vi "Send Cmd To Stimulator_v0.1.vi"(0 "Stimulator In":T2={"Log File In"=refnum, "Stimulator In"="", "Stimulator Mode"="", "Log Data"=FALSE, "Doublet/Triplet  Interval"=0.0, "Stim Frequency"=40.0, "N-Factor"=0, "Active Channels"=[TRUE, TRUE, TRUE, TRUE, TRUE], "Low-Frequency Channels"=[FALSE, FALSE, FALSE, FALSE, FALSE], "Stimulator State"=enum."Closed", "Mode Array"=[], "Current Array"=[], "Pulse Duration Array"=[], "VISA Timeout"=50}, 1 "Command":T1, 3 "error in (no error)":errorcluster) -> (4 "Numeric Response":u8, 5 "Stimulator Out":T2={"Log File In"=refnum, "Stimulator In"="", "Stimulator Mode"="", "Log Data"=FALSE, "Doublet/Triplet  Interval"=0.0, "Stim Frequency"=40.0, "N-Factor"=0, "Active Channels"=[TRUE, TRUE, TRUE, TRUE, TRUE], "Low-Frequency Channels"=[FALSE, FALSE, FALSE, FALSE, FALSE], "Stimulator State"=enum."Closed", "Mode Array"=[], "Current Array"=[], "Pulse Duration Array"=[], "VISA Timeout"=50}, 6 "Command":T1, 7 "Log Entry":string, 8 "error out":errorcluster)   [LabVIEW 2019]
uses:
  Controls/Stimulator Cluster.ctl
  Controls/Stimulator Mode.ctl
  Version 2/Data Type Defs/Pulse Mode (array).ctl
  Controls/Stim Current Array.ctl
  Controls/Pulse Duration Array.ctl
  Bits Library/Get Bit (U8).vi
  Bits Library/Change Bit (U8).vi
  Bits Library/Bits.lvlib
panel:
  out "Write Error":errorcluster
  out "Bytes written":u32
  out "Bytes read":u32
  out "Read Error":errorcluster
  out "resulting string":string
  out "string":string
  out "hex integer string":string
  out "Number Out":u8 format="%.0x"
  out "appended array":bool[](array[boolean])
  out "element":u8 format="%0d"
  out "unsigned byte array 2":u8[](array[numeric]) format="%08b"
  out "Bytes available":u32
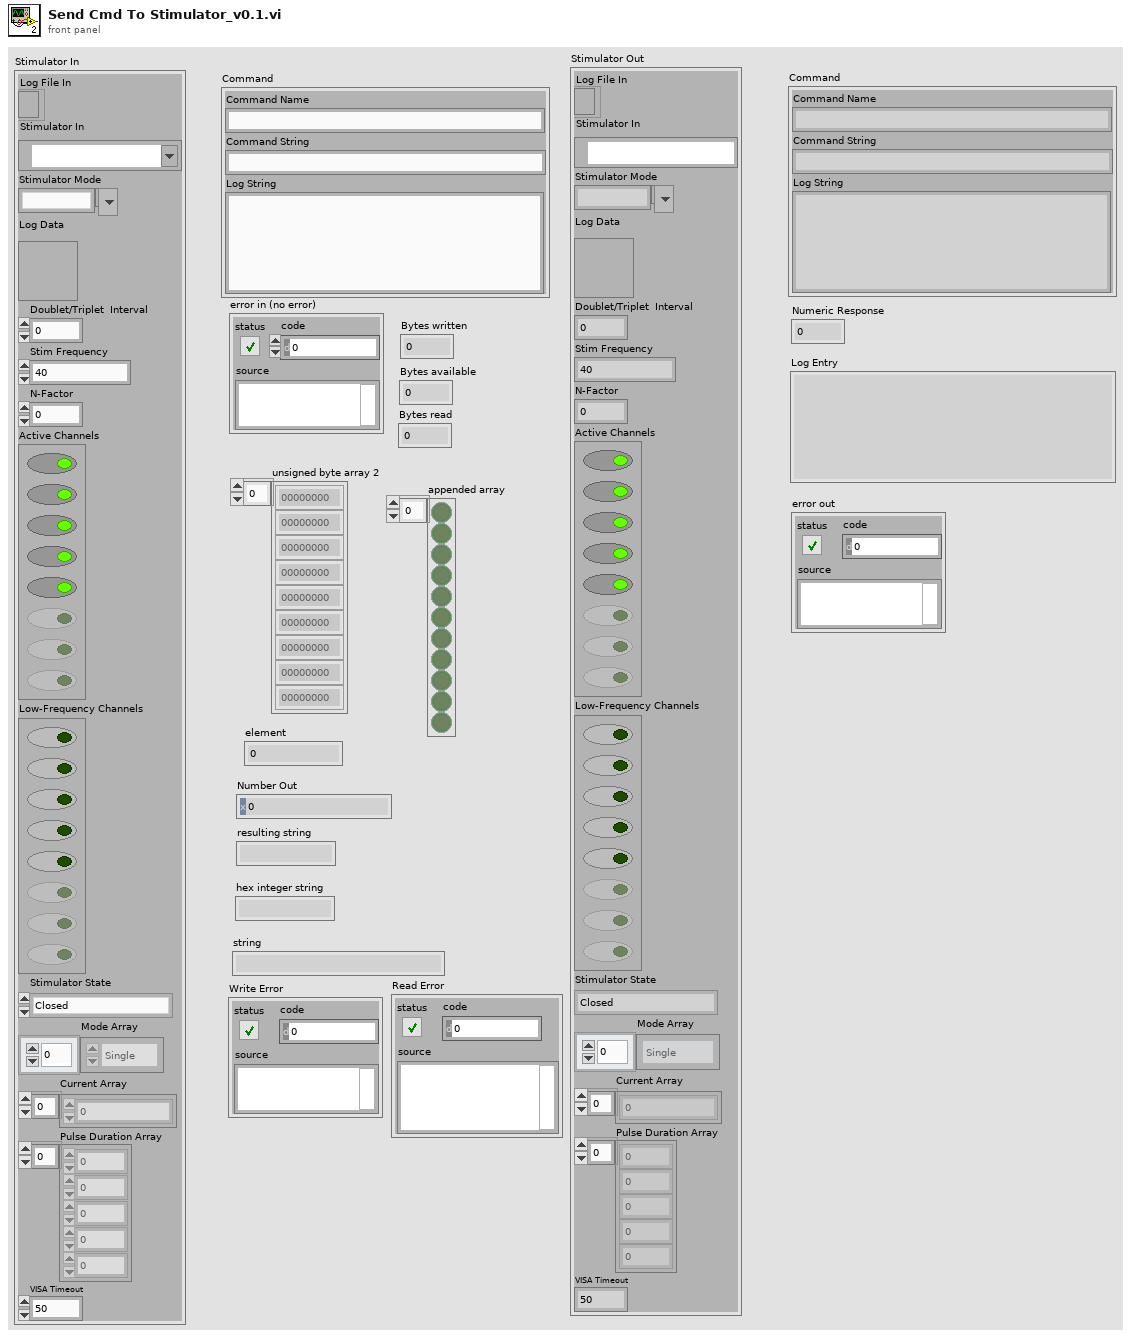
[diagram p1: front panel]
types:
  T1 = cluster{"Command Name":string, "Command String":string, "Log String":string}
  T2 = typedef "Stimulator Cluster.ctl" = cluster{"Log File In":refnum<file>, "Stimulator In":refnum<visa-resource-name>, "Stimulator Mode":T3, "Log Data":bool, "Doublet/Triplet  Interval":dbl, "Stim Frequency":dbl, "N-Factor":u8, "Active Channels":bool[], "Low-Frequency Channels":bool[], "Stimulator State":enum16{"Closed", "Open", "Initialized", "Stimulating"}, "Mode Array":T4, "Current Array":T5, "Pulse Duration Array":T6, "VISA Timeout":u32}
  T3 = typedef "Stimulator Mode.ctl" = string
  T4 = typedef "Pulse Mode (array).ctl" = enum16{"Single", "Doublet", "Triplet"}[]
  T5 = typedef "Stim Current Array.ctl" = u8[]
  T6 = typedef "Pulse Duration Array.ctl" = u32[]
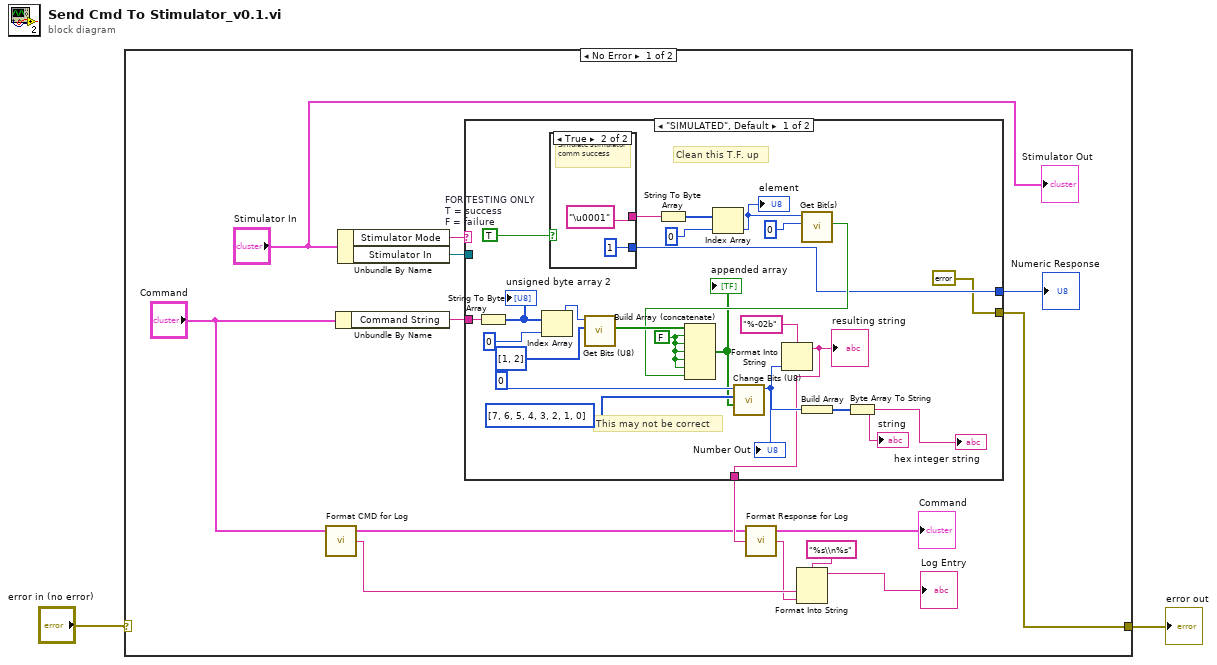
[diagram p0: block diagram]
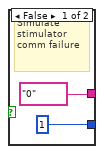
[diagram p2: hidden frame]
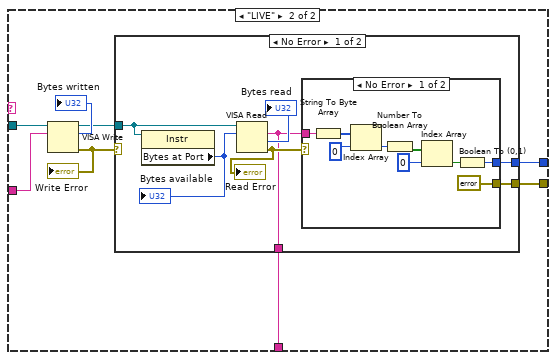
[diagram p3: hidden frame]
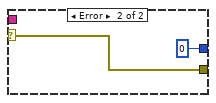
[diagram p4: hidden frame]
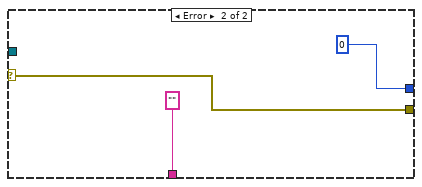
[diagram p5: hidden frame]
diagram:
  n1 = case shown="No Error" "error in (no error)" {
    selector: "error in (no error)" -> [_ w74]
    tunnel: [w10 w74] -> w1
    frame No Error {
      n2 = call "Format CMD for Log.vi"("Command"="Command") -> ("Stim CMD for Log"=w6:string, "Command"=w8:T1)  [unwired: 2 in, 1 out]
      n3 = Unbundle By Name("Command") -> ("Command String"=w13:string)
      n4 = Unbundle By Name("Stimulator In") -> ("Stimulator Mode"=w16:T3, "Stimulator In"=w11:refnum<visa-resource-name>)
      n5 = case shown="\"SIMULATED\", Default" w16 {
        tunnel: w13 -> [w39 w52]
        tunnel: [w19 w48] -> w12
        tunnel: w11 -> [_ w47]
        tunnel: [errorcluster {"status"=FALSE, "code"=0, "source"=""} ("error IO") w46] -> w10
        tunnel: [w18 w45] -> w9
        frame "SIMULATED", Default {
          w30 = FALSE
          w40 = TRUE  # FOR TESTING ONLY T = success F = failure
          # "Clean this T.F. up"
          # "This may not be correct"
          n6 = String To Byte Array(string=w39) -> (unsigned byte array=w38:u8[])
          "unsigned byte array 2" <- w38
          n7 = Index Array(array=w38, index=0) -> (element=w36:u8)
          n8 = case shown="True" w40 {
            tunnel: ["0" "\u0001"] -> w32
            tunnel: [1 1] -> w19
            frame False {
              # "Simulate stimulator comm failure"
            }
            frame True {
              # "Simulate stimulator comm success"
            }
          }
          n9 = call "Get Bits (U8).vi"("Bits"=u8[] [1, 2], "Number"=w36) -> ("Values"=w31:bool[])  [unwired: 8 in, 1 out]
          n10 = String To Byte Array(string=w32) -> (unsigned byte array=w34:u8[])
          n11 = Index Array(array=w34, index=0) -> (element=w27:u8)
          "element" <- w27
          n12 = call-poly "Get Bit(s).vi"("Bit"=u8 0, "Number"=w27) -> ("Value"=w25:bool)  [unwired: 8 in, 1 out]
          n13 = Build Array (concatenate)(w31, w30, w30, w30, w30, w30, w25) -> (w21:bool[])
          "appended array" <- w21
          n14 = call "Change Bits (U8).vi"("Values"=w21, "Bits"=u8[] [7, 6, 5, 4, 3, 2, 1, 0], "Number"=u8 0) -> ("Number Out"=w20:u8)  [unwired: 8 in]
          "Number Out" <- w20
          n15 = Format Into String(format string="%-02b", w20) -> (resulting string=w18:string)  [unwired: 2 in, 1 out]
          "resulting string" <- w18
          n16 = Build Array(w20) -> (w24:u8[])
          n17 = Byte Array To String(unsigned byte array=w24) -> (string=→"hex integer string" →"string":string)
        }
        frame "LIVE" {
          n18 = VISA Write(VISA resource name=w47, write buffer=w52) -> (VISA resource name out=w49:refnum<visa-resource-name>, return count=→"Bytes written":u32, error out=w50:errorcluster)  [unwired: 1 in]
          "Write Error" <- w50
          n19 = case shown="No Error" w50 {
            selector: w50 -> [_ w73]
            tunnel: w49 -> [w58 _]
            tunnel: [w56 u8 0] -> w48
            tunnel: [w54 w73] -> w46
            tunnel: [w53 "" ("read buffer")] -> w45
            frame No Error {
              n20 = property class="Instr"(reference=w58) -> ("Bytes at Port"=w57:u32)  [unwired: 1 in, 2 out]
              "Bytes available" <- w57
              n21 = VISA Read(VISA resource name=w58, byte count=w57) -> (read buffer=w53:string, return count=→"Bytes read":u32, error out=w59:errorcluster)  [unwired: 1 in, 1 out]
              "Read Error" <- w59
              n22 = case shown="No Error" w59 {
                selector: w59 -> [_ w70]
                tunnel: [w60 u8 0] -> w56
                tunnel: w53 -> [w66 _]
                tunnel: [errorcluster {"status"=FALSE, "code"=0, "source"=""} ("error IO") w70] -> w54
                frame No Error {
                  n23 = String To Byte Array(string=w66) -> (unsigned byte array=w68:u8[])
                  n24 = Index Array(array=w68, index=0) -> (element=w64:u8)
                  n25 = Number To Boolean Array(number=w64) -> (Boolean array=w63:bool[])
                  n26 = Index Array(array=w63, index=0) -> (element=w61:bool)
                  n27 = Boolean To (0,1)(Boolean=w61) -> (0, 1=w60:i16)
                }
                frame Error {
                }
              }
            }
            frame Error {
            }
          }
        }
      }
      "Numeric Response" <- w12
      n28 = call "Format Response for Log.vi"("Response"=w9, "Command"=w8) -> ("Stim RSP for Log"=w3:string, "Command"=→"Command":T1)  [unwired: 1 in, 1 out]
      n29 = Format Into String(format string="%s\\n%s", w6, w3) -> (resulting string=→"Log Entry":string)  [unwired: 2 in, 1 out]
      "Stimulator Out" <- "Stimulator In"
    }
    frame Error {
    }
  }
  "error out" <- w1
